vi "Event 3 Mouse Down.vi"(4 "User Parameter":variant, 5 "Event Data":cluster{"sender":refnum<k24>, "e":refnum<k24>}, 6 "Control Ref":refnum<k24>, 7 "Event Common Data":T1) -> ()   [LabVIEW 2014]
uses:
  C:/Robotic Systems/Products/Surveyor/Software/Ground Station/Data/Mapping DLL/GMap.NET.WindowsForms.dll
  Data/Mapping DLL/GMap.NET.WindowsForms.dll
  System.Windows.Forms
  Controls/GMap Mouse States.ctl
  FGVs/GMap Mouse State/Methods/SET Mouse State.vi
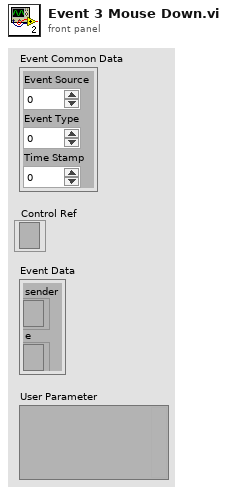
[diagram p1: front panel]
types:
  T1 = cluster{"Event Source":i32, "Event Type":u32, "Time Stamp":u32}
  T2 = typedef "GMap Mouse States.ctl" = enum16{"Mouse Down", "Mouse Up"}
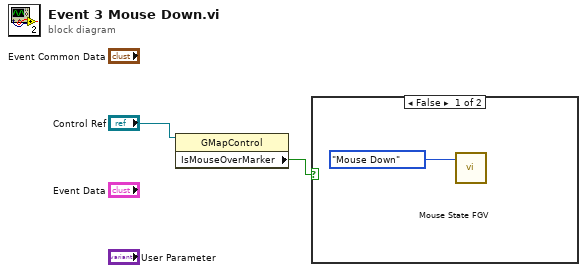
[diagram p0: block diagram]
diagram:
  n1 = property class="GMapControl"(reference="Control Ref") -> ("IsMouseOverMarker"=w1:bool)  [unwired: 1 in, 2 out]
  n2 = case shown="False" w1 {
    frame False {
      n3 = call-poly "Mouse State FGV.vi"("Mouse State In"=GMap_Mouse_States."Mouse Down") -> ()  [unwired: 10 in, 1 out]
    }
    frame True {
    }
  }
